vi "_ADC_ Signal Quantization.vi"(6 "ADC Internal Parametes":T1={"ADC Resolution"=enum."8", "ADC Gain Error"=0.0, "ADC Offset Error"=0.0, "ADC Sampling Frequency Jitter"=0.0, "ADC Sampling Frequency"=44100.0}, 7 "Supply Parameters":T2={"ADC Supply Ripple Frequency"=10.0, "Gen Wave Sampling Frequency"=0.0, "ADC Neg Supply Ripple Amplitude"=0.0, "ADC Neg Supply Offset"=0.0, "ADC Pos Supply Ripple Amplitude"=0.0, "ADC Pos Supply Offset"=0.0, "ADC Supply Diff Noise Amplitude"=0.0}, 9 "Input Wave":waveform(dbl)) -> (3 "Output Wave":waveform(dbl))   [LabVIEW 2014]
uses:
  Ctls/_ADC_ Supply Variables.ctl
  Ctls/_ADC_ Internal Variables.ctl
  <vilib>/Utility/miscctls.llb/LVFormatAndPrecisionTypeDef.ctl
panel:
  out "XY Graph":cluster{dbl[], dbl[]}[](graph)
  out "Least Num of Bits":dbl
  out "Measured LSB":dbl
  out "Calculated LSB":dbl=1.0
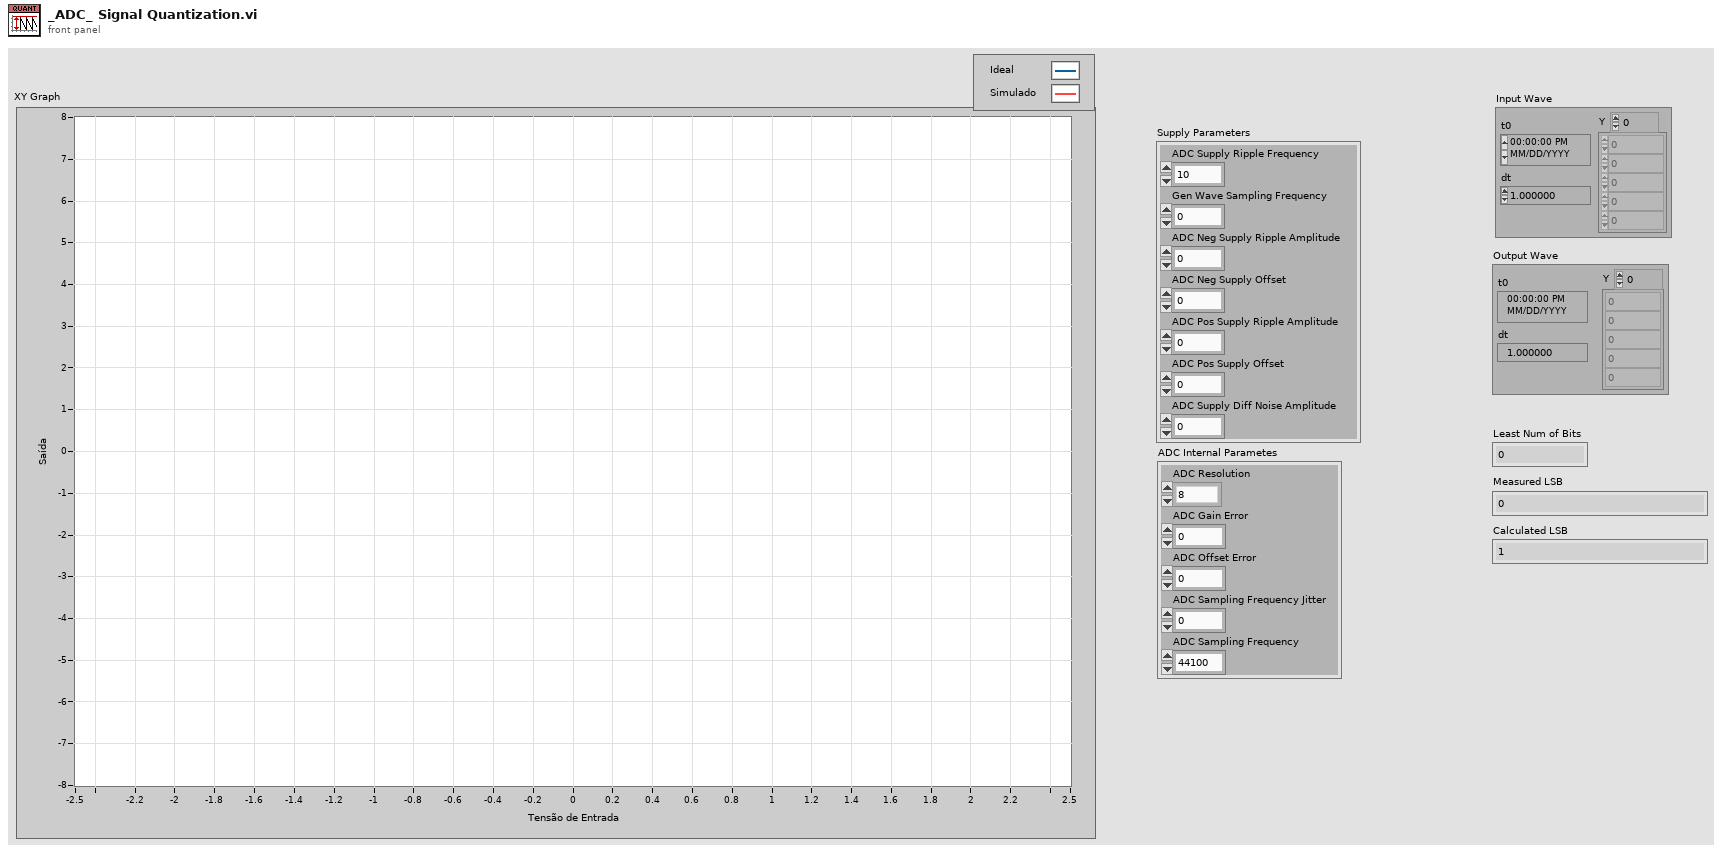
[diagram p1: front panel]
types:
  T1 = typedef "_ADC_ Internal Variables.ctl" = cluster{"ADC Resolution":enum16{"0", "1", "2", "3", "4", "5", "6", "7", "8", "9", "10", "11", "12", "13", "14", "15", "16", "17", "18", "19", "20", "21", "22", "23", "24", "25", "26", "27", "28", "29", "30", "31", "32"}, "ADC Gain Error":dbl, "ADC Offset Error":dbl, "ADC Sampling Frequency Jitter":dbl, "ADC Sampling Frequency":dbl}
  T2 = typedef "_ADC_ Supply Variables.ctl" = cluster{"ADC Supply Ripple Frequency":dbl, "Gen Wave Sampling Frequency":dbl, "ADC Neg Supply Ripple Amplitude":dbl, "ADC Neg Supply Offset":dbl, "ADC Pos Supply Ripple Amplitude":dbl, "ADC Pos Supply Offset":dbl, "ADC Supply Diff Noise Amplitude":dbl}
  T3 = typedef "LVFormatAndPrecisionTypeDef.ctl" = cluster{"Format":u8, "Precision":u8}
  T4 = enum16{"Vetor Naive", "Vector LSB", "Point-by-Point Naive", "Point-by-Point Delta"}
  T5 = enum16{"0", "1", "2", "3", "4", "5", "6", "7", "8", "9", "10", "11", "12", "13", "14", "15", "16", "17", "18", "19", "20", "21", "22", "23", "24", "25", "26", "27", "28", "29", "30", "31", "32"}
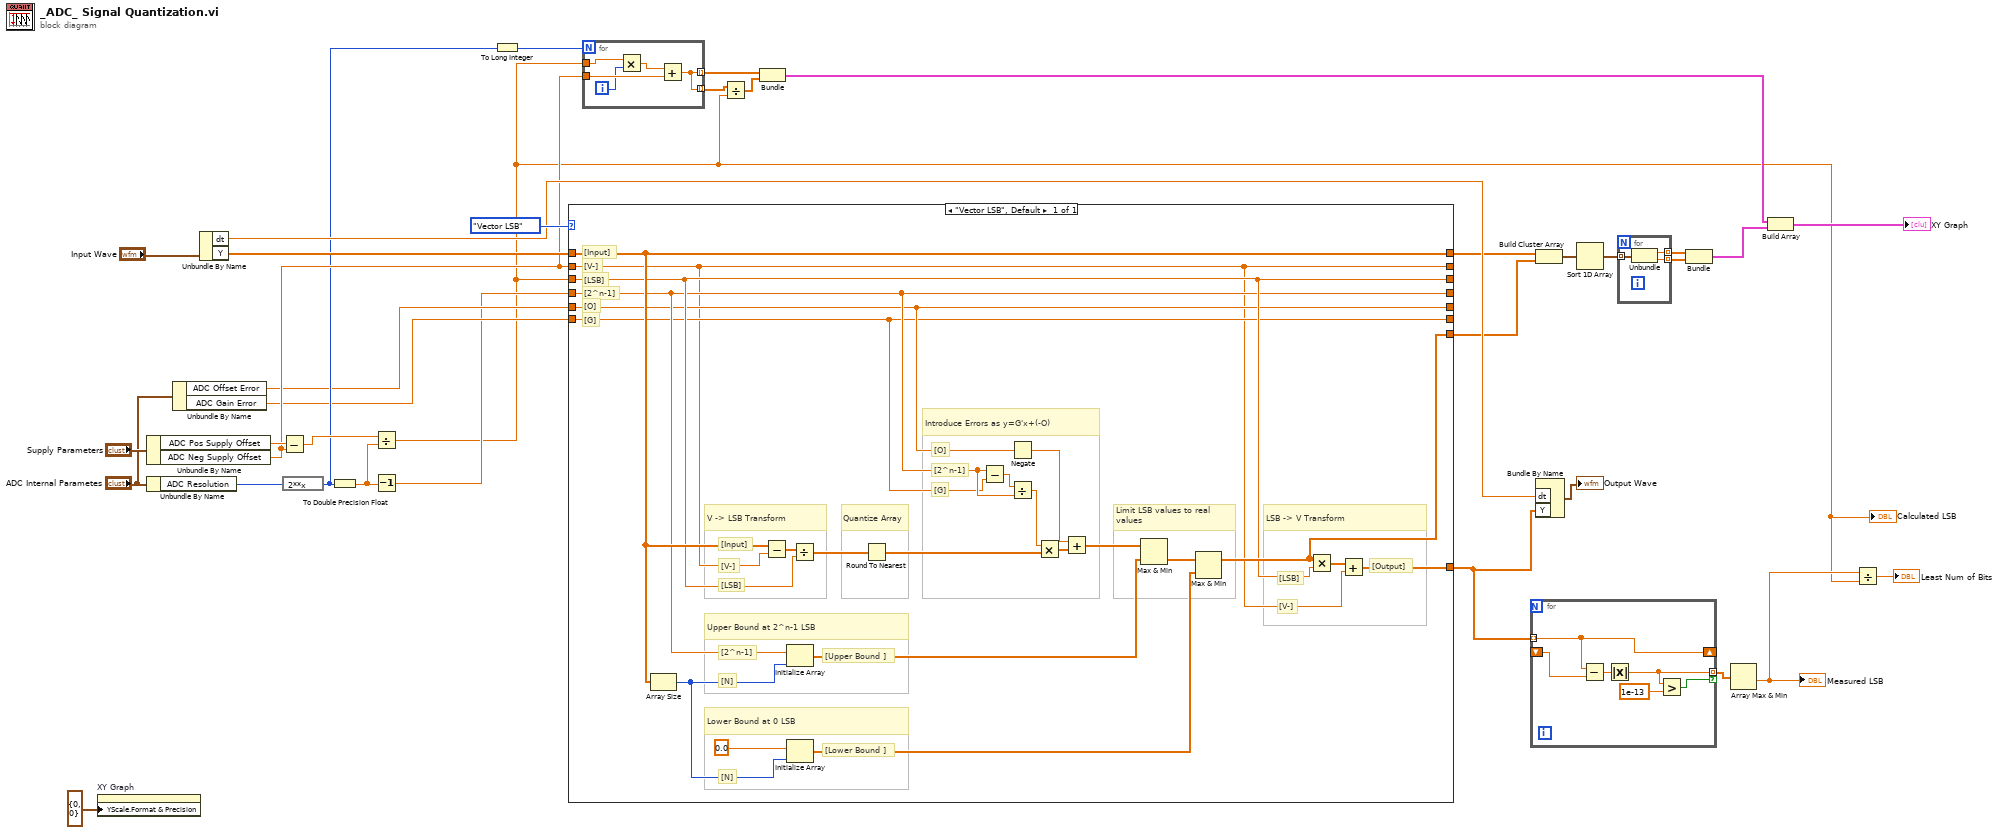
[diagram p0: block diagram]
diagram:
  n1 = property on="XY Graph" class="XYGraph (strict)"("YScale.Format & Precision"=T3 {"Format"=0, "Precision"=0} ("Y Scale.Display Format")) -> ()  [unwired: 2 in, 2 out]
  n2 = Unbundle By Name("Supply Parameters") -> ("ADC Pos Supply Offset"=w30:dbl, "ADC Neg Supply Offset"=w17:dbl)
  n3 = Unbundle By Name("ADC Internal Parametes") -> ("ADC Resolution"=w19:T5)
  n4 = Unbundle By Name("ADC Internal Parametes") -> ("ADC Offset Error"=w6:dbl, "ADC Gain Error"=w5:dbl)
  n5 = Unbundle By Name("Input Wave") -> ("dt"=w27:dbl, "Y"=w23:dbl[])
  n6 = Subtract(x=w30, y=w17) -> (x-y=w29:dbl)
  n7 = expression code="2**x"(w19) -> (w16:T5)
  n8 = To Double Precision Float(number=w16) -> (double precision float=w7:dbl)
  n9 = Divide(x=w29, y=w7) -> (x/y=w3:dbl)
  "Calculated LSB" <- w3
  n10 = Decrement(x=w7) -> (x-1=w4:dbl)
  n11 = To Long Integer(number=w16) -> (32bit integer=w15:i32)
  n12 = case shown="\"Vector LSB\", Default" T4."Vector LSB" ("Quantization Mode") {
    tunnel: w23 -> [w45]
    tunnel: [w54] -> w21
    tunnel: [w36] -> w28
    tunnel: w3 -> [w42]
    tunnel: w17 -> [w37]
    tunnel: w4 -> [w41]
    tunnel: [w45] -> w8
    tunnel: w6 -> [w40]
    tunnel: w5 -> [w39]
    tunnel: [w37] -> _
    tunnel: [w42] -> _
    tunnel: [w41] -> _
    tunnel: [w40] -> _
    tunnel: [w39] -> _
    frame "Vector LSB", Default {
      # "[Output]"
      # "[V-]"
      # "[LSB]"
      # "LSB -> V Transform"
      # "Limit LSB values to real \nvalues"
      # "[G]"
      # "[O]"
      # "[2^n-1]"
      # "[G]"
      # "[O]"
      # "[Input]"
      # "[V-]"
      # "[LSB]"
      # "[2^n-1]"
      # "[Input]"
      # "[V-]"
      # "[LSB]"
      # "[N]"
      # "[N]"
      # "[Lower Bound ]"
      # "[Upper Bound ]"
      # "[2^n-1]"
      # "Introduce Errors as y=G'x+(-O)"
      # "Quantize Array"
      # "V -> LSB Transform"
      # "Lower Bound at 0 LSB"
      # "Upper Bound at 2^n-1 LSB"
      n13 = Array Size(array=w45) -> (size(s)=w43:i32)
      n14 = Subtract(x=w45, y=w37) -> (x-y=w44:dbl[])
      n15 = Initialize Array(w41, w43) -> (w56:dbl[])
      n16 = Initialize Array(0.0 ("element"), w43) -> (w53:dbl[])
      n17 = Divide(x=w44, y=w42) -> (x/y=w57:dbl[])
      n18 = Round To Nearest(number=w57) -> (nearest integer value=w50:dbl[])
      n19 = Subtract(x=w41, y=w39) -> (x-y=w48:dbl)
      n20 = Negate(x=w40) -> (-x=w46:dbl)
      n21 = Divide(x=w48, y=w41) -> (x/y=w47:dbl)
      n22 = Multiply(x=w47, y=w50) -> (x*y=w49:dbl[])
      n23 = Add(x=w46, y=w49) -> (x+y=w55:dbl[])
      n24 = Max & Min(x=w55, y=w56) -> (min(x,y)=w51:dbl[])  [unwired: 1 out]
      n25 = Max & Min(x=w51, y=w53) -> (max(x,y)=w54:dbl[])  [unwired: 1 out]
      n26 = Multiply(x=w54, y=w42) -> (x*y=w38:dbl[])
      n27 = Add(x=w38, y=w37) -> (x+y=w36:dbl[])
    }
  }
  n28 = for {
    N: w15 -> [_]
    tunnel: w17 -> [w62]
    tunnel: w3 -> [w60]
    tunnel: [w58] -> w18 mode=indexing
    tunnel: [w58] -> w9 mode=indexing
    i -> [w59]
    n29 = Multiply(x=w60, y=w59) -> (x*y=w61:dbl)
    n30 = Add(x=w61, y=w62) -> (x+y=w58:dbl)
  }
  n31 = Divide(x=w9, y=w3) -> (x/y=w10:dbl[])
  n32 = Bundle(w18, w10) -> (w13:cluster{dbl[], dbl[]})  [unwired: 1 in]
  n33 = for {
    tunnel: w28 -> [w65] mode=indexing
    shift-right: [w65] -> _
    shift-left: _ -> [w66]
    tunnel: [w64] -> w34 mode=indexing if=w63
    n34 = Subtract(x=w65, y=w66) -> (x-y=w67:dbl)
    n35 = Absolute Value(x=w67) -> (abs(x)=w64:dbl)
    n36 = Greater?(x=w64, y=1e-13) -> (0:w63:bool)
  }
  n37 = Bundle By Name("dt"=w27, "Y"=w28) -> (→"Output Wave":waveform(dbl))  [unwired: 1 in]
  n38 = Build Cluster Array(w8, w21) -> (w25:cluster{dbl, dbl}[])
  n39 = Sort 1D Array(array=w25) -> (sorted array=w24:cluster{dbl, dbl}[])
  n40 = for {
    tunnel: w24 -> [w71] mode=indexing
    tunnel: [w70] -> w22 mode=indexing
    tunnel: [w69] -> w20 mode=indexing
    n41 = Unbundle(w71) -> (w70:dbl, w69:dbl)
  }
  n42 = Bundle(w22, w20) -> (w14:cluster{dbl[], dbl[]})  [unwired: 1 in]
  n43 = Array Max & Min(array=w34) -> (min value=w33:dbl)  [unwired: 3 out]
  "Measured LSB" <- w33
  n44 = Build Array(w13, w14) -> (→"XY Graph":cluster{dbl[], dbl[]}[])
  n45 = Divide(x=w33, y=w3) -> (x/y=→"Least Num of Bits":dbl)
